vi "dataconverter.vi"(11 "appended array":waveform(dbl)[](array[waveform])) -> (1 "XY Graph":cluster{dbl[], dbl[]}(graph), 3 "transposed array":dbl[][](array[numeric]))   [LabVIEW 2020]
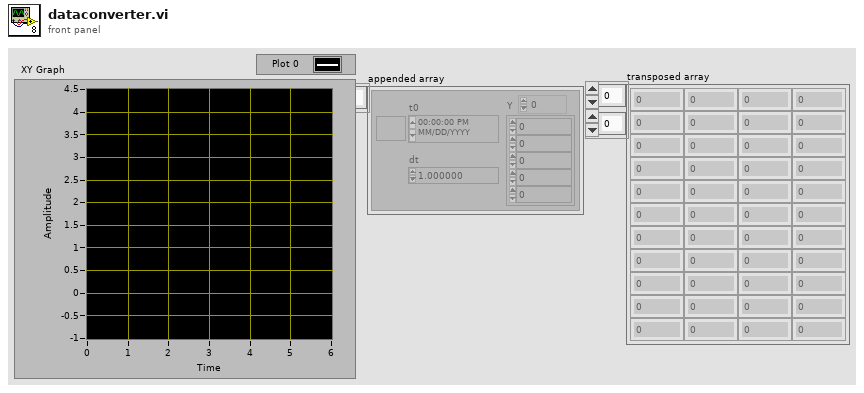
[diagram p1: front panel]
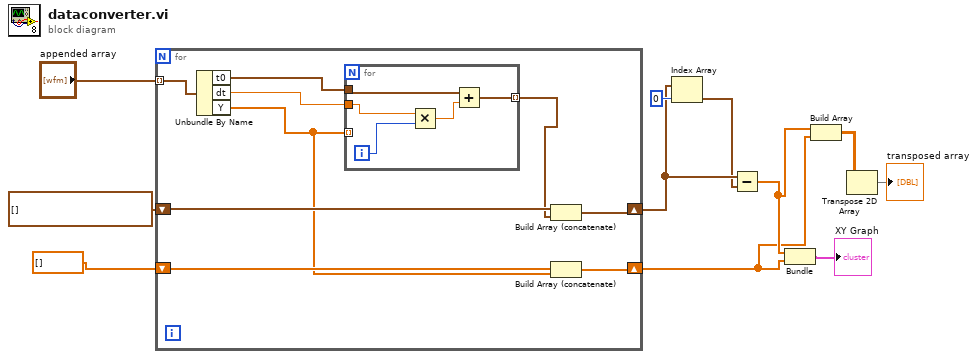
[diagram p0: block diagram]
diagram:
  n1 = for {
    tunnel: "appended array" -> [w20] mode=indexing
    shift-right: [w17] -> w7
    shift-left: timestamp[] [] -> [w15]
    shift-right: [w16] -> w3
    shift-left: dbl[] [] -> [w14]
    n2 = Unbundle By Name(w20) -> ("t0"=w19:timestamp, "dt"=w18:dbl, "Y"=w12:dbl[])
    n3 = for {
      tunnel: w12 -> [_] mode=indexing
      tunnel: w19 -> [w23]
      tunnel: w18 -> [w25]
      tunnel: [w21] -> w13 mode=indexing
      i -> [w24]
      n4 = Multiply(x=w25, y=w24) -> (x*y=w22:dbl)
      n5 = Add(x=w23, y=w22) -> (x+y=w21:timestamp)
    }
    n6 = Build Array (concatenate)(w15, w13) -> (w17:timestamp[])
    n7 = Build Array (concatenate)(w14, w12) -> (w16:dbl[])
  }
  n8 = Index Array(array=w7, index=0) -> (element=w6:timestamp)
  n9 = Subtract(x=w7, y=w6) -> (x-y=w4:dbl[])
  n10 = Bundle(w4, w3) -> (→"XY Graph":cluster{dbl[], dbl[]})  [unwired: 1 in]
  n11 = Build Array(w4, w3) -> (w2:dbl[][])
  n12 = Transpose 2D Array(2D array=w2) -> (transposed array=→"transposed array":dbl[][])
